vi "UpdateSetting.vi"(8 "error in (no error)":errorcluster, 10 "Setting":u32, 11 "Controller in":refnum<class "Controller.lvclass">) -> (0 "error out":errorcluster, 3 "Controller out":refnum<class "Controller.lvclass">)   [LabVIEW 2020, in "Page1.lvlib" / "Controller.lvclass"]
uses:
  Controller.lvclass
  Controller.lvclass/Controller.ctl
  Model/Model/Model.lvclass
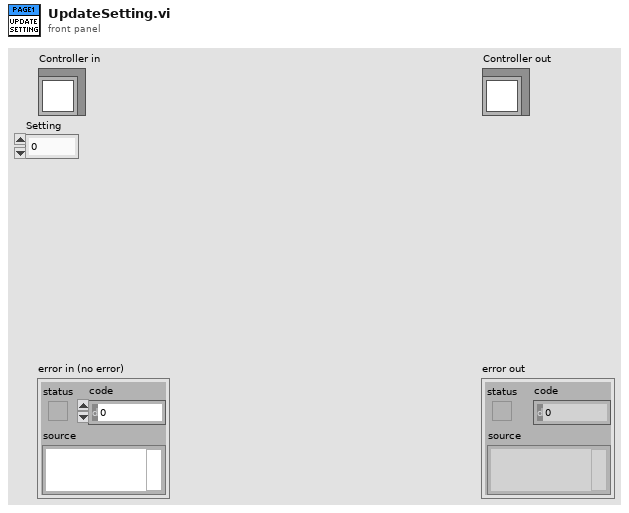
[diagram p1: front panel]
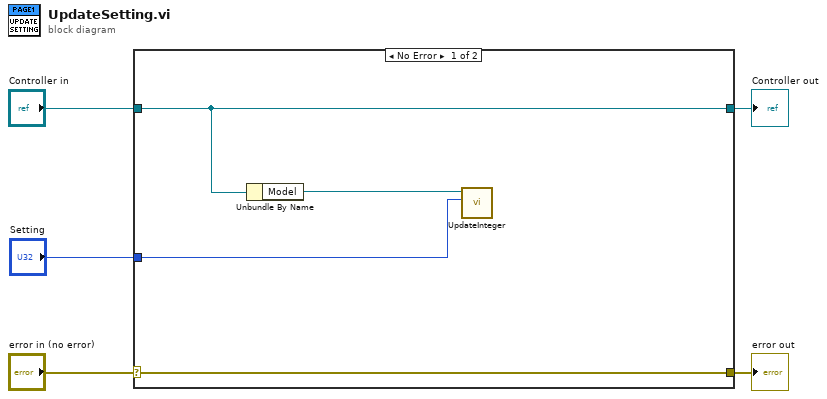
[diagram p0: block diagram]
diagram:
  n1 = case shown="No Error" "error in (no error)" {
    selector: "error in (no error)" -> [w7 w11]
    tunnel: [w7 w11] -> w4
    tunnel: [w9 w10] -> w2
    tunnel: "Controller in" -> [w9 w10]
    tunnel: "Setting" -> [w8 _]
    frame No Error {
      n2 = Unbundle By Name(w9) -> ("Model"=w6:refnum<class "Model.lvclass">)
      n3 = call "UpdateInteger.vi"("Integer"=w8, "Model in"=w6) -> ()  [unwired: 8 in, 2 out]
    }
    frame Error {
    }
  }
  "error out" <- w4
  "Controller out" <- w2
